vi "Project Sync Tools Mod.vi"() -> ()   [LabVIEW 2019]
uses:
  Project Sync Tools/TypeDefs/BuildSpec Source.ctl
  Project Sync Tools/Project Sync Tools.lvclass
panel:
  in  "Project Path":path
  out "Errors":errorcluster
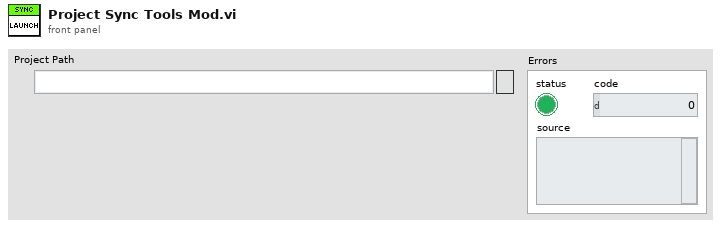
[diagram p1: front panel]
types:
  T1 = typedef "Project Sync Tools.lvclass/BuildSpec Source.ctl" = cluster{"Source Library":string, "Source Folder":string, "Apply Inclusion":bool}
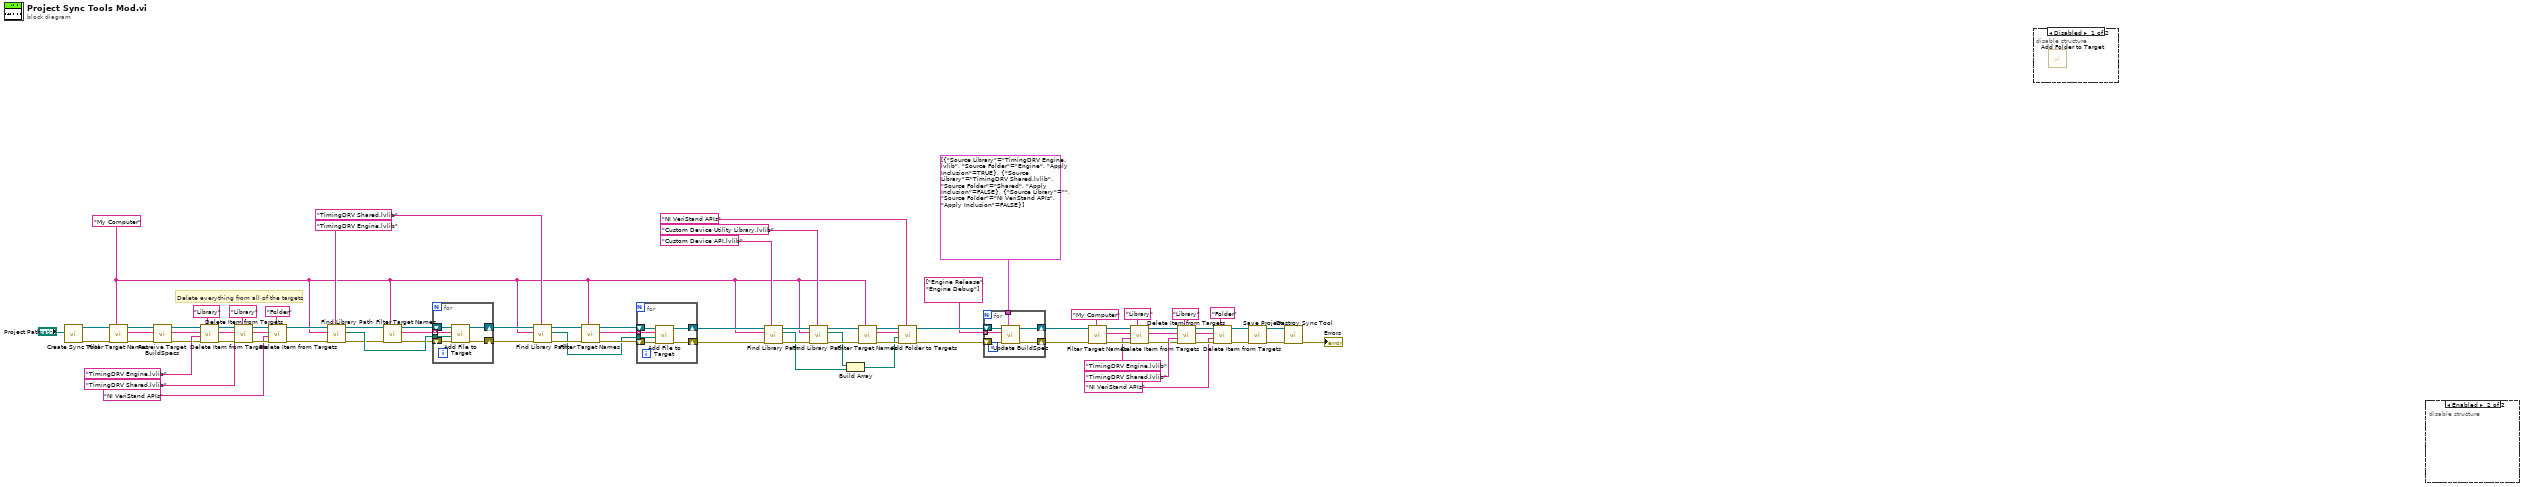
[diagram p0: block diagram]
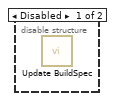
[diagram p3: hidden frame]
diagram:
  w24 = "My Computer" ("Target Name")
  # "Delete everything from all of the targets"
  n1 = call "Create Sync Tool.vi"("File Path Control"="Project Path") -> ("error out"=w57:errorcluster, "CD Build Tools out"=w58:refnum<class "Project Sync Tools.lvclass">)  [unwired: 9 in]
  n2 = call "Filter Target Names.vi"("Target Name"=w24, "error in (no error)"=w57, "Project Sync Tools in"=w58) -> ("error out"=w23:errorcluster, "Filtered Names"=w21:string[], "Project Sync Tools out"=w22:refnum<class "Project Sync Tools.lvclass">)  [unwired: 6 in]
  n3 = call "Retreive Target BuildSpecs.vi"("error in (no error)"=w23, "Target Names in"=w21, "Project Sync Tools in"=w22) -> ("error out"=w18:errorcluster, "Target Names out"=w19:string[], "Project Sync Tools out"=w20:refnum<class "Project Sync Tools.lvclass">)  [unwired: 6 in]
  n4 = call "Delete Item from Targets.vi"("Type"="Library", "error in (no error)"=w18, "Item Name"="TimingDRV Engine.lvlib" ("Library Name"), "Target Names in"=w19, "Project Sync Tools in"=w20) -> ("error out"=w73:errorcluster, "Target Names out"=w66:string[], "Project Sync Tools out"=w74:refnum<class "Project Sync Tools.lvclass">)  [unwired: 4 in]
  n5 = call "Delete Item from Targets.vi"("Type"="Library", "error in (no error)"=w73, "Item Name"="TimingDRV Shared.lvlib" ("Library Name"), "Target Names in"=w66, "Project Sync Tools in"=w74) -> ("error out"=w70:errorcluster, "Target Names out"=w65:string[], "Project Sync Tools out"=w69:refnum<class "Project Sync Tools.lvclass">)  [unwired: 4 in]
  n6 = call "Delete Item from Targets.vi"("Type"="Folder", "error in (no error)"=w70, "Item Name"="NI VeriStand APIs", "Target Names in"=w65, "Project Sync Tools in"=w69) -> ("error out"=w63:errorcluster, "Project Sync Tools out"=w64:refnum<class "Project Sync Tools.lvclass">)  [unwired: 4 in, 1 out]
  n7 = call "Find Library Path.vi"("Library Name"="TimingDRV Engine.lvlib", "error in (no error)"=w63, "Target Name"=w24, "Project Sync Tools in"=w64) -> ("error out"=w62:errorcluster, "Library Path"=w77:path, "Project Sync Tools out"=w45:refnum<class "Project Sync Tools.lvclass">)  [unwired: 4 in, 1 out]
  n8 = call "Filter Target Names.vi"("Target Name"=w24, "error in (no error)"=w62, "Project Sync Tools in"=w45) -> ("error out"=w60:errorcluster, "Filtered Names"=w59:string[], "Project Sync Tools out"=w61:refnum<class "Project Sync Tools.lvclass">)  [unwired: 6 in]
  n9 = for {
    shift-right: [w86] -> w54
    shift-left: w60 -> [w88]
    shift-right: [w85] -> w53
    shift-left: w61 -> [w87]
    tunnel: w77 -> [w84]
    tunnel: w59 -> [w83] mode=indexing
    n10 = call "Add File to Target.vi"("error in (no error)"=w88, "Flie Path"=w84, "Target Name"=w83, "Project Sync Tools in"=w87) -> ("error out"=w86:errorcluster, "Project Sync Tools out"=w85:refnum<class "Project Sync Tools.lvclass">)  [unwired: 6 in]
  }
  n11 = call "Find Library Path.vi"("Library Name"="TimingDRV Shared.lvlib", "error in (no error)"=w54, "Target Name"=w24, "Project Sync Tools in"=w53) -> ("error out"=w51:errorcluster, "Library Path"=w46:path, "Project Sync Tools out"=w50:refnum<class "Project Sync Tools.lvclass">)  [unwired: 4 in, 1 out]
  n12 = call "Filter Target Names.vi"("Target Name"=w24, "error in (no error)"=w51, "Project Sync Tools in"=w50) -> ("error out"=w47:errorcluster, "Filtered Names"=w48:string[], "Project Sync Tools out"=w49:refnum<class "Project Sync Tools.lvclass">)  [unwired: 6 in]
  n13 = for {
    shift-right: [w92] -> w40
    shift-left: w47 -> [w94]
    shift-right: [w91] -> w39
    shift-left: w49 -> [w93]
    tunnel: w46 -> [w90]
    tunnel: w48 -> [w89] mode=indexing
    n14 = call "Add File to Target.vi"("error in (no error)"=w94, "Flie Path"=w90, "Target Name"=w89, "Project Sync Tools in"=w93) -> ("error out"=w92:errorcluster, "Project Sync Tools out"=w91:refnum<class "Project Sync Tools.lvclass">)  [unwired: 6 in]
  }
  n15 = call "Find Library Path.vi"("Library Name"="Custom Device API.lvlib", "error in (no error)"=w40, "Target Name"=w24, "Project Sync Tools in"=w39) -> ("error out"=w42:errorcluster, "Library Path"=w35:path, "Project Sync Tools out"=w41:refnum<class "Project Sync Tools.lvclass">)  [unwired: 4 in, 1 out]
  n16 = call "Find Library Path.vi"("Library Name"="Custom Device Utility Library.lvlib", "error in (no error)"=w42, "Target Name"=w24, "Project Sync Tools in"=w41) -> ("error out"=w38:errorcluster, "Library Path"=w36:path, "Project Sync Tools out"=w37:refnum<class "Project Sync Tools.lvclass">)  [unwired: 4 in, 1 out]
  n17 = Build Array(w36, w35) -> (w27:path[])
  n18 = call "Filter Target Names.vi"("Target Name"=w24, "error in (no error)"=w38, "Project Sync Tools in"=w37) -> ("error out"=w31:errorcluster, "Filtered Names"=w29:string[], "Project Sync Tools out"=w30:refnum<class "Project Sync Tools.lvclass">)  [unwired: 6 in]
  n19 = call "Add Folder to Targets.vi"("Folder Name"="NI VeriStand APIs" ("Name"), "error in (no error)"=w31, "Content Paths"=w27, "Target Names"=w29, "Project Sync Tools in"=w30) -> ("error out"=w25:errorcluster, "Project Sync Tools out"=w26:refnum<class "Project Sync Tools.lvclass">)  [unwired: 5 in]
  n20 = for {
    tunnel: T1[] [{"Source Library"="TimingDRV Engine.lvlib", "Source Folder"="Engine", "Apply Inclusion"=TRUE}, {"Source Library"="TimingDRV Shared.lvlib", "Source Folder"="Shared", "Apply Inclusion"=FALSE}, {"Source Library"="", "Source Folder"="NI VeriStand APIs", "Apply Inclusion"=FALSE}] ("BuildSpec Sources") -> [w98]
    shift-right: [w99] -> w55
    shift-left: w26 -> [w97]
    shift-right: [w100] -> w56
    shift-left: w25 -> [w96]
    tunnel: string[] ["Engine Release", "Engine Debug"] -> [w95] mode=indexing
    n21 = call "Update BuildSpec.vi"("BuildSpec Sources"=w98, "error in (no error)"=w96, "Target Build Spec"=w95, "CD Build Tools in"=w97) -> ("error out"=w100:errorcluster, "CD Build Tools out"=w99:refnum<class "Project Sync Tools.lvclass">)  [unwired: 6 in]
  }
  n22 = call "Filter Target Names.vi"("Target Name"="My Computer", "error in (no error)"=w56, "Project Sync Tools in"=w55) -> ("error out"=w16:errorcluster, "Filtered Names"=w14:string[], "Project Sync Tools out"=w15:refnum<class "Project Sync Tools.lvclass">)  [unwired: 6 in]
  n23 = call "Delete Item from Targets.vi"("Type"="Library", "error in (no error)"=w16, "Item Name"="TimingDRV Engine.lvlib" ("Library Name"), "Target Names in"=w14, "Project Sync Tools in"=w15) -> ("error out"=w3:errorcluster, "Target Names out"=w2:string[], "Project Sync Tools out"=w4:refnum<class "Project Sync Tools.lvclass">)  [unwired: 4 in]
  n24 = call "Delete Item from Targets.vi"("Type"="Library", "error in (no error)"=w3, "Item Name"="TimingDRV Shared.lvlib" ("Library Name"), "Target Names in"=w2, "Project Sync Tools in"=w4) -> ("error out"=w9:errorcluster, "Target Names out"=w5:string[], "Project Sync Tools out"=w8:refnum<class "Project Sync Tools.lvclass">)  [unwired: 4 in]
  n25 = call "Delete Item from Targets.vi"("Type"="Folder", "error in (no error)"=w9, "Item Name"="NI VeriStand APIs", "Target Names in"=w5, "Project Sync Tools in"=w8) -> ("error out"=w33:errorcluster, "Project Sync Tools out"=w32:refnum<class "Project Sync Tools.lvclass">)  [unwired: 4 in, 1 out]
  n26 = call "Save Project.vi"("error in (no error)"=w33, "Project Sync Tools in"=w32) -> ("error out"=w80:errorcluster, "Project Sync Tools out"=w79:refnum<class "Project Sync Tools.lvclass">)  [unwired: 8 in]
  n27 = call "Destroy Sync Tool.vi"("error in (no error)"=w80, "CD Build Tools in"=w79) -> ("error out"=→"Errors":errorcluster)  [unwired: 9 in]
  n28 = disable-structure shown="Disabled" {
    frame Disabled {
      n29 = call "Add Folder to Target.vi"() -> ()  [unwired: 9 in, 3 out]
    }
    frame Enabled {
    }
  }
  n30 = disable-structure shown="Enabled" {
    frame Disabled {
      n31 = call "Update BuildSpec.vi"() -> ()  [unwired: 10 in, 2 out]
    }
    frame Enabled {
    }
  }
